vi "Image Processing Main.vi"() -> ()   [LabVIEW 2009]
uses:
  <vilib>/vision/driver/NI_Vision_Acquisition_Software.lvlib
  <vilib>/vision/driver/IMAQdx.llb/IMAQdx Acquisition Mode.ctl
  <vilib>/userDefined/High Color/IMAQdx.ctl
panel:
  out "Sick array":i32[](array[numeric])
  out "x-y":u32
  in  "stop":bool
  out "Right Camera Input":T1(plugin-control)
  out "Left Camera Input":T1(plugin-control)
  out "Right Camera Output":T1(plugin-control)
  out "Left Camera Output":T1(plugin-control)
  in  "IMAQdx Session Right":T2="cam1" caption="Session In"
  in  "IMAQdx Session Left":T2="cam0" caption="Session In"
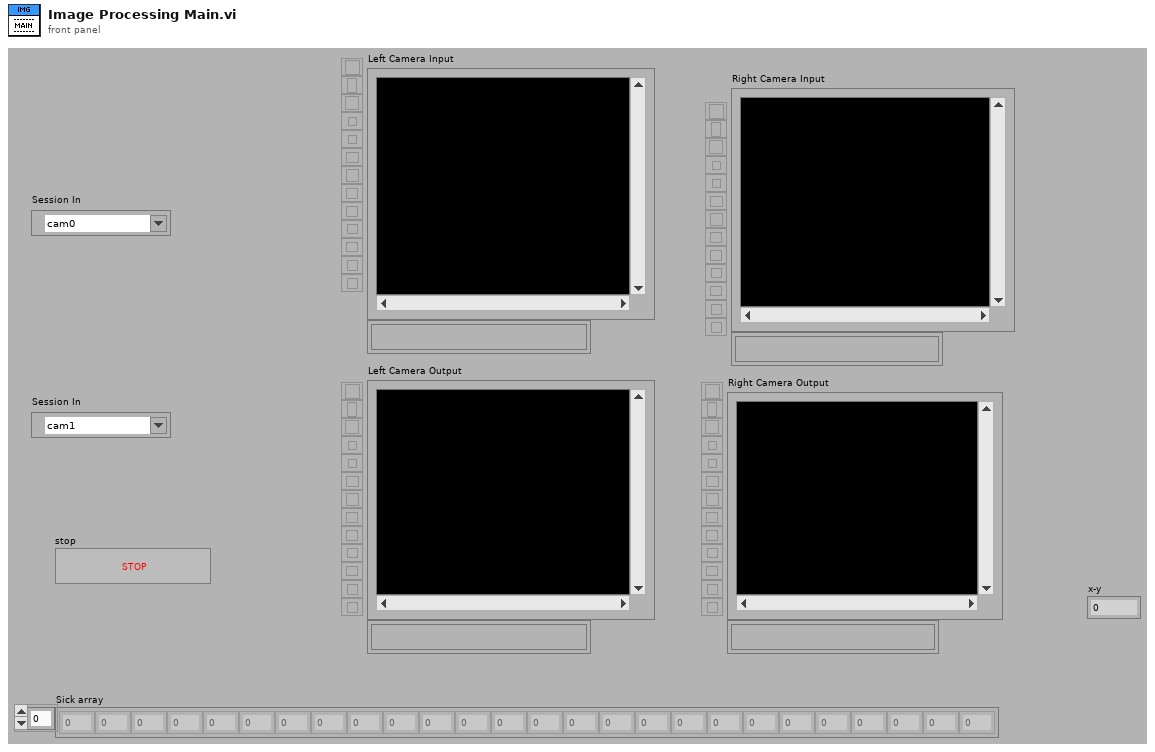
[diagram p1: front panel]
types:
  T1 = typedef "IMAQ Image.ctl" = refnum<image>
  T2 = typedef "IMAQdx.ctl" = refnum<k21>
  T3 = typedef "NI_Vision_Acquisition_Software.lvlib/IMAQdx Acquisition Mode.ctl" = enum32{"One Shot", "Continuous"}
  T4 = typedef "Image Type" = u32
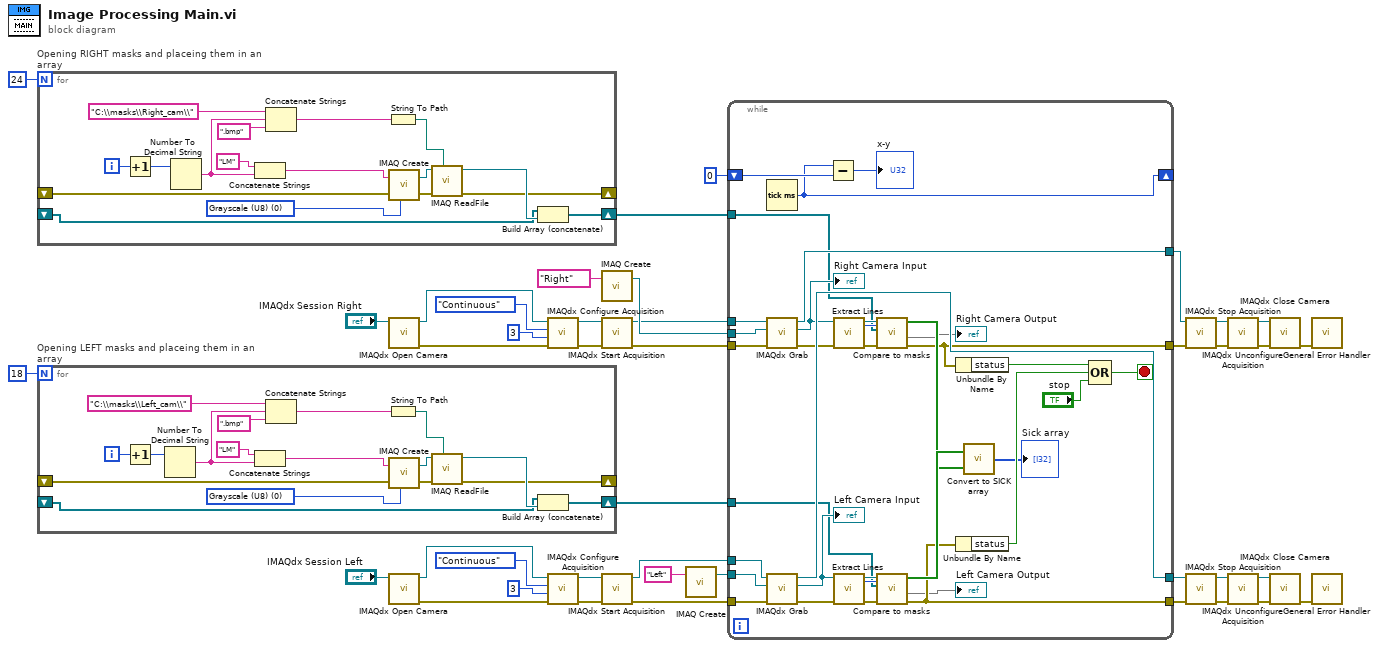
[diagram p0: block diagram]
diagram:
  n1 = for "Opening RIGHT masks and placeing them in an array" {
    N: 24 -> [_]
    shift-right: [w52] -> w3
    shift-left: _ -> [w51]
    shift-right: [w50] -> _
    shift-left: _ -> [w49]
    i -> [w56]
    w54 = T4 0 items=["Grayscale (U8)", "Grayscale (I16)", "Grayscale (SGL)", "Complex (CSG)", "RGB (U32)", "HSL (U32)", "RGB (U64)", "Grayscale (U16)"] ("Image Type")
    n2 = Increment(x=w56) -> (x+1=w55:i32)
    n3 = Number To Decimal String(number=w55) -> (decimal integer string=w46:string)  [unwired: 1 in]
    n4 = Concatenate Strings("LM" ("element"), w46) -> (w42:string)
    n5 = Concatenate Strings("C:\\masks\\Right_cam\\", w46, ".bmp") -> (w43:string)
    n6 = String To Path(string=w43) -> (path=w44:path)
    n7 = call "IMAQ Create"("Image Name"=w42, "Image Type"=w54, "error in (no error)"=w49) -> ("New Image"=w57:T1, "error out"=w58:errorcluster)  [unwired: 2 in]
    n8 = call "IMAQ ReadFile"("File Path"=w44, "error in (no error)"=w58, "Image"=w57) -> ("error out"=w50:errorcluster, "Image Out"=w53:T1)  [unwired: 4 in, 3 out]
    n9 = Build Array (concatenate)(w51, w53) -> (w52:T1[])
  }
  n10 = for "Opening LEFT masks and placeing them in an array" {
    N: 18 -> [_]
    shift-right: [w69] -> w1
    shift-left: _ -> [w68]
    shift-right: [w67] -> _
    shift-left: _ -> [w66]
    i -> [w73]
    w71 = T4 0 items=["Grayscale (U8)", "Grayscale (I16)", "Grayscale (SGL)", "Complex (CSG)", "RGB (U32)", "HSL (U32)", "RGB (U64)", "Grayscale (U16)"] ("Image Type")
    n11 = Increment(x=w73) -> (x+1=w72:i32)
    n12 = Number To Decimal String(number=w72) -> (decimal integer string=w63:string)  [unwired: 1 in]
    n13 = Concatenate Strings("LM" ("element"), w63) -> (w59:string)
    n14 = Concatenate Strings("C:\\masks\\Left_cam\\", w63, ".bmp") -> (w60:string)
    n15 = String To Path(string=w60) -> (path=w61:path)
    n16 = call "IMAQ Create"("Image Name"=w59, "Image Type"=w71, "error in (no error)"=w66) -> ("New Image"=w74:T1, "error out"=w75:errorcluster)  [unwired: 2 in]
    n17 = call "IMAQ ReadFile"("File Path"=w61, "error in (no error)"=w75, "Image"=w74) -> ("error out"=w67:errorcluster, "Image Out"=w70:T1)  [unwired: 4 in, 3 out]
    n18 = Build Array (concatenate)(w68, w70) -> (w69:T1[])
  }
  n19 = call <vilib>:"IMAQdx Open Camera.vi"("Session In"="IMAQdx Session Right") -> ("error out"=w28:errorcluster, "Session Out"=w29:T2)  [unwired: 2 in, 7 out]
  n20 = call <vilib>:"IMAQdx Open Camera.vi"("Session In"="IMAQdx Session Left") -> ("error out"=w36:errorcluster, "Session Out"=w35:T2)  [unwired: 2 in, 7 out]
  n21 = call <vilib>:"IMAQdx Configure Acquisition.vi"("error in"=w28, "Number of Buffers"=u32 3, "Continuous?"=IMAQdx_Acquisition_Mode."Continuous", "Session In"=w29) -> ("error out"=w27:errorcluster, "Session Out"=w30:T2)  [unwired: 1 in, 5 out]
  n22 = call <vilib>:"IMAQdx Configure Acquisition.vi"("error in"=w36, "Number of Buffers"=u32 3, "Continuous?"=IMAQdx_Acquisition_Mode."Continuous", "Session In"=w35) -> ("error out"=w37:errorcluster, "Session Out"=w34:T2)  [unwired: 1 in, 5 out]
  n23 = call "IMAQ Create"("Image Name"="Right") -> ("New Image"=w40:T1)  [unwired: 4 in, 1 out]
  n24 = call <vilib>:"IMAQdx Start Acquisition.vi"("error in"=w27, "Session In"=w30) -> ("error out"=w25:errorcluster, "Session Out"=w26:T2)  [unwired: 8 out]
  n25 = call <vilib>:"IMAQdx Start Acquisition.vi"("error in"=w37, "Session In"=w34) -> ("error out"=w32:errorcluster, "Session Out"=w33:T2)  [unwired: 8 out]
  n26 = call "IMAQ Create"("Image Name"="Left") -> ("New Image"=w39:T1)  [unwired: 4 in, 1 out]
  n27 = while {
    tunnel: w33 -> [w109]
    tunnel: w39 -> [w108]
    tunnel: w25 -> [w107]
    tunnel: w26 -> [w106]
    tunnel: w32 -> [w105]
    tunnel: w40 -> [w104]
    tunnel: [w103] -> w11
    tunnel: [w102] -> w18
    tunnel: [w84] -> w10
    tunnel: [w83] -> w17
    shift-right: [w96] -> _
    shift-left: u32 0 -> [w97]
    tunnel: w3 -> [w77]
    tunnel: w1 -> [w76]
    stop <- w98 stop-if-true
    n28 = Tick Count (ms)() -> (millisecond timer value=w96:u32)
    n29 = call <vilib>:"IMAQdx Grab.vi"("error in"=w107, "Image In"=w104, "Session In"=w106) -> ("error out"=w93:errorcluster, "Image Out"=w94:T1, "Session Out"=w102:T2)  [unwired: 5 in, 1 out]
    "Right Camera Input" <- w94
    n30 = call <vilib>:"IMAQdx Grab.vi"("error in"=w105, "Image In"=w108, "Session In"=w109) -> ("error out"=w91:errorcluster, "Image Out"=w92:T1, "Session Out"=w103:T2)  [unwired: 5 in, 1 out]
    "Left Camera Input" <- w92
    n31 = Subtract(x=w96, y=w97) -> (x-y=→"x-y":u32)
    n32 = call "Extract Lines.vi"("error in (no error)"=w93, "Image Src"=w94) -> ("error out"=w88:errorcluster, "Image Out"=w79:T1, "Extraction mode"=w89:i32)  [unwired: 6 in, 1 out]
    n33 = call "Extract Lines.vi"("error in (no error)"=w91, "Image Src"=w92) -> ("error out"=w87:errorcluster, "Image Out"=w78:T1, "Extraction mode"=w90:i32)  [unwired: 6 in, 1 out]
    n34 = call "Compare to masks.vi"("Number of Particles1"=w89, "error in (no error)"=w88, "Mask array"=w77, "Image Src"=w79) -> ("Final error out"=w83:errorcluster, 1:→"Right Camera Output", "Marked Regions"=w85:bool[])  [unwired: 5 in]
    n35 = call "Compare to masks.vi"("Number of Particles1"=w90, "error in (no error)"=w87, "Mask array"=w76, "Image Src"=w78) -> ("Final error out"=w84:errorcluster, 1:→"Left Camera Output", "Marked Regions"=w86:bool[])  [unwired: 5 in]
    n36 = Unbundle By Name(w83) -> ("status"=w101:bool)
    n37 = Unbundle By Name(w84) -> ("status"=w100:bool)
    n38 = call "Convert to SICK array.vi"("Right regions"=w85, "Left regions"=w86) -> ("Sick array"=→"Sick array":i32[])  [unwired: 1 in]
    n39 = Compound Arithmetic op=OR(w101, w100, "stop") -> (w98:bool)
  }
  n40 = call <vilib>:"IMAQdx Stop Acquisition.vi"("error in"=w17, "Session In"=w18) -> ("error out"=w21:errorcluster, "Session Out"=w20:T2)  [unwired: 8 out]
  n41 = call <vilib>:"IMAQdx Stop Acquisition.vi"("error in"=w10, "Session In"=w11) -> ("error out"=w14:errorcluster, "Session Out"=w15:T2)  [unwired: 8 out]
  n42 = call <vilib>:"IMAQdx Unconfigure Acquisition.vi"("error in"=w21, "Session In"=w20) -> ("error out"=w22:errorcluster, "Session Out"=w23:T2)  [unwired: 8 out]
  n43 = call <vilib>:"IMAQdx Unconfigure Acquisition.vi"("error in"=w14, "Session In"=w15) -> ("error out"=w13:errorcluster, "Session Out"=w12:T2)  [unwired: 8 out]
  n44 = call <vilib>:"IMAQdx Close Camera.vi"("error in"=w22, "Session In"=w23) -> ("error out"=w19:errorcluster)  [unwired: 9 out]
  n45 = call <vilib>:"IMAQdx Close Camera.vi"("error in"=w13, "Session In"=w12) -> ("error out"=w16:errorcluster)  [unwired: 9 out]
  n46 = call <vilib>:"General Error Handler.vi"("error in (no error)"=w19) -> ()  [unwired: 1 in, 14 out]
  n47 = call <vilib>:"General Error Handler.vi"("error in (no error)"=w16) -> ()  [unwired: 1 in, 14 out]
